vi "ComputeBlocks.vi"(7 "MD5":refnum<class "MD5.lvclass">, 10 "blocks queue":refnum<queue>) -> (2 "hash":u8[](array[numeric]) format="%02x")   [LabVIEW 2013, in "MD5.lvlib" / "MD5.lvclass"]
doc: "This VI contains the core of the MD5 algorithm."
uses:
  MD5.lvclass
  Data-vector.ctl
  K-Vector.vi
  S-Vector.vi
  F.vi
  G.vi
  H.vi
  I.vi
  T-Vector.vi
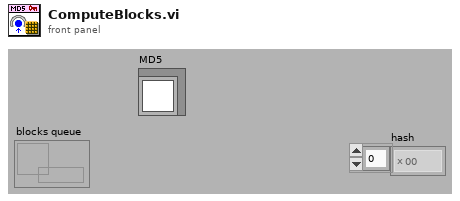
[diagram p1: front panel]
types:
  T1 = typedef "MD5.lvlib/MD5.lvclass/Data-vector.ctl" = cluster{"Data[ ]":u8[], "end":bool}
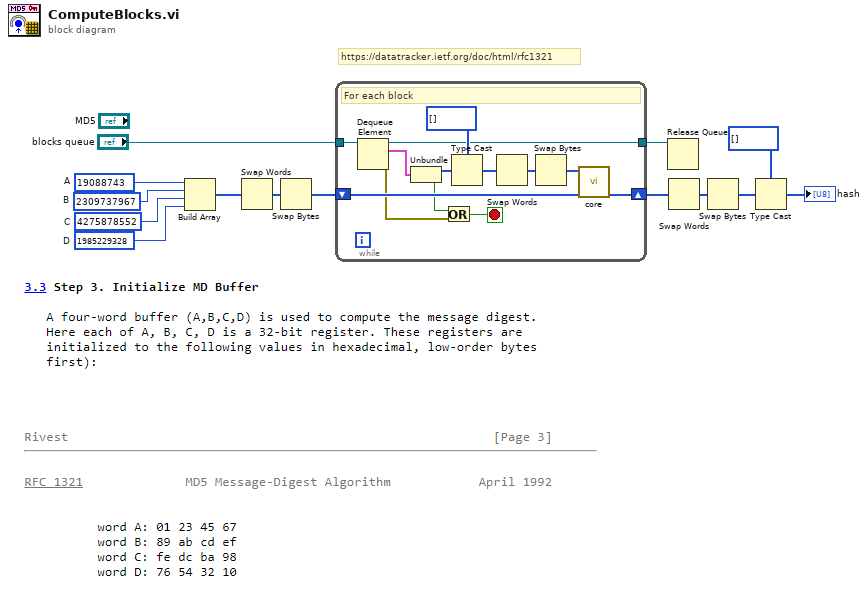
[diagram p0: block diagram]
diagram:
  w10 = u32 1985229328  # D
  w11 = u32 4275878552  # C
  w12 = u32 2309737967  # B
  w13 = u32 19088743  # A
  # "https://datatracker.ietf.org/doc/html/rfc1321"
  n1 = Build Array(w13, w12, w11, w10) -> (w8:u32[])
  n2 = Swap Words(1:w8) -> (0:w3:u32[])
  n3 = Swap Bytes(anything=w3) -> (byte swapped=w7:u32[])
  n4 = while {
    shift-right: [w26] -> w6
    shift-left: w7 -> [w27]
    tunnel: "blocks queue" -> [w25]
    tunnel: [w15] -> w1
    stop <- w16 stop-if-true
    # "For each block"
    n5 = Dequeue Element(queue=w25) -> (queue out=w15:refnum<queue>, element=w24:T1, error out=w22:errorcluster)  [unwired: 2 in, 1 out]
    n6 = Unbundle(w24) -> ("Data[ ]"=w23:u8[], "end"=w21:bool)
    n7 = Or(x=w21, y=w22) -> (x .or. y?=w16:bool)
    n8 = Type Cast(type=u32[] [] ("U32"), x=w23) -> (*(type *) &x=w17:u32[])
    n9 = Swap Words(1:w17) -> (0:w20:u32[])
    n10 = Swap Bytes(anything=w20) -> (byte swapped=w19:u32[])
    n11 = call "core.vi"("ABCD in"=w27, "M[ ]"=w19) -> ("ABCD out"=w26:u32[])  [unwired: 9 in]
  }
  n12 = Release Queue(queue=w1) -> ()  [unwired: 2 in, 3 out]
  n13 = Swap Words(1:w6) -> (0:w4:u32[])
  n14 = Swap Bytes(anything=w4) -> (byte swapped=w5:u32[])
  n15 = Type Cast(type=u8[] [], x=w5) -> (*(type *) &x=→"hash":u8[])
